vi "InputOneFrame.vi"(8 "error in (no error)":errorcluster caption="错误输入（无错误）", 9 "pstInputFrameInfo In":T1, 10 "handle":u64, 11 "pData":u8[](array[numeric])) -> (0 "error out":errorcluster caption="错误输出", 1 "pstInputFrameInfo Out":T1, 2 "handle out":u64, 3 "function return":i32)   [LabVIEW 2011, in "MvCameraControl.lvlib"]
doc: "MV_LV_API int __stdcall SaveImage(MV_SAVE_IMAGE_PARAM* pSaveParam);"
uses:
  MvCameraControl.lvlib
  x86/MvCameraPatch.dll
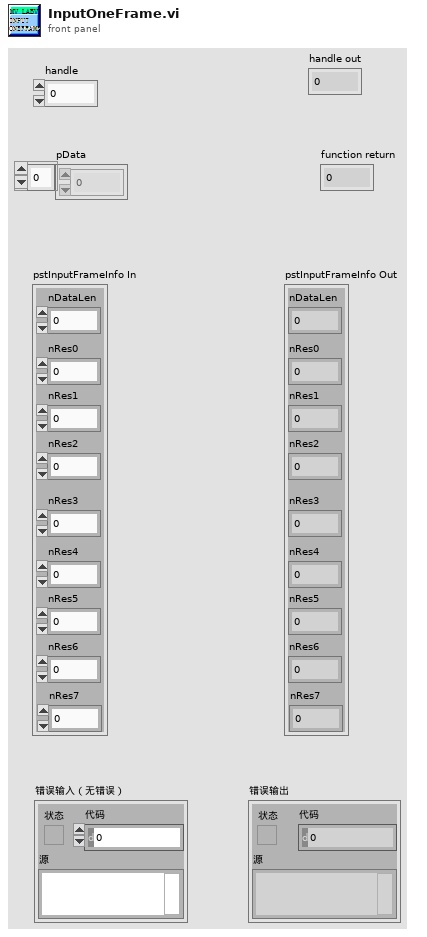
[diagram p1: front panel]
types:
  T1 = cluster{"nDataLen":u32, "nRes0":u32, "nRes1":u32, "nRes2":u32, "nRes3":u32, "nRes6":u32, "nRes5":u32, "nRes4":u32, "nRes7":u32}
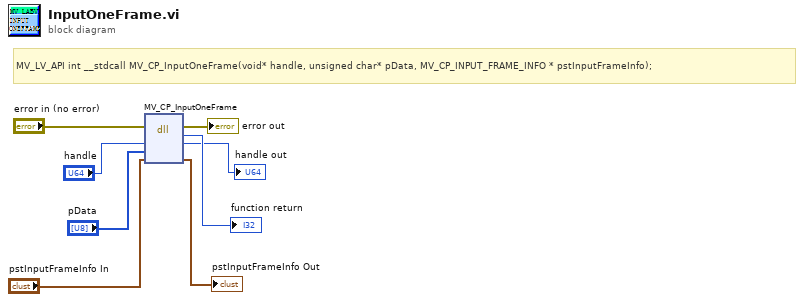
[diagram p0: block diagram]
diagram:
  # "MV_LV_API int __stdcall MV_CP_InputOneFrame(void* handle, unsigned char* pData, MV_CP_INPUT_FRAME_INFO * pstInputFrameInfo);"
  n1 = dll-call lib="F:/SVN/SDK/Release/MVS/Samples/Labview/MvLVLib/x86/MvCameraPatch.dll" fn="MV_CP_InputOneFrame"(error in="error in (no error)", "handle"="handle", "pData"="pData", "pstInputFrameInfo"="pstInputFrameInfo In") -> (error out=→"error out":errorcluster, "返回类型"=→"function return":i32, "handle"=→"handle out":u64, "pstInputFrameInfo"=→"pstInputFrameInfo Out":T1)  [unwired: 3 in, 1 out]
